vi "CICDPathConfigLV2.vi"(6 "Set? (F)":bool, 11 "CICD Path Config In":T1) -> (3 "CICD Path Config Out":T1)   [LabVIEW 2023, in "Reusables.lvlib"]
uses:
  Reusables.lvlib
  Typedefs/CICDPathConfigs.ctl
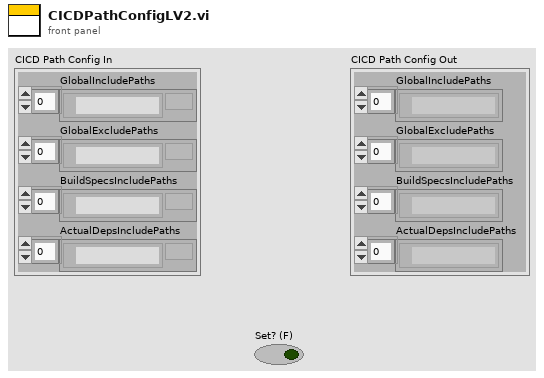
[diagram p1: front panel]
types:
  T1 = typedef "Reusables.lvlib/CICDPathConfigs.ctl" = cluster{"GlobalIncludePaths":path[], "GlobalExcludePaths":path[], "BuildSpecsIncludePaths":path[], "ActualDepsIncludePaths":path[]}
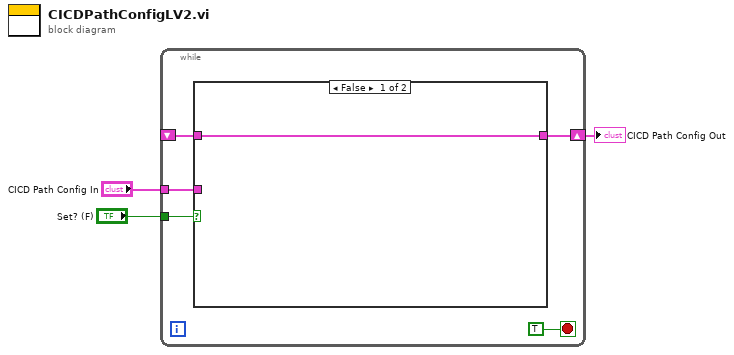
[diagram p0: block diagram]
diagram:
  n1 = while {
    tunnel: "Set? (F)" -> [w7]
    tunnel: "CICD Path Config In" -> [w6]
    shift-right: [w5] -> w1
    shift-left: _ -> [w4]
    stop <- TRUE stop-if-true
    n2 = case shown="False" w7 {
      tunnel: w6 -> [_ w10]
      tunnel: [w9 w10] -> w5
      tunnel: w4 -> [w9 _]
      frame False {
      }
      frame True {
      }
    }
  }
  "CICD Path Config Out" <- w1
